vi "Define Columns.vi"() -> (2 "Column Definitions":T1[](array[typedef]) {"MinWidth" min=2 step=1; "AutoSizeMode" items=["None"=1, "ColumnHeader"=2, "AllCellsExceptHeader"=4, "AllCells"=6, "DisplayedCellsExceptHeader"=8, "DisplayedCells"=10, "Fill"=16]; "FillWeight" min=1 max=100})   [LabVIEW 2013, in "Modbus Module editor node.lvclass"]
uses:
  Modbus Module editor node.lvclass
  <vilib>/NI/DCAF Table API/Column/Column Descriptor.ctl
  <vilib>/NI/DCAF Table API/Column/Column Type.ctl
  <vilib>/NI/Tag Bus/tag/Data Type.ctl
  <vilib>/NI/DCAF Table API/Table Manager/Call Back Ref Type Def.ctl
  <vilib>/NI/DCAF/Tag Editor Core/Configuration Editor/Classes/Engine Parent/Engine Parent Editor Node.lvclass
  <vilib>/NI/DCAF/Tag Editor Core/Configuration Editor/Classes/Module editor node/module editor node.lvclass
  <vilib>/NI/DCAF Table API/Column/Column.lvclass
  <vilib>/NI/DCAF Table API/Mapping Column/Mapping Column.lvclass
  <vilib>/NI/DCAF Table API/String Column/String Column.lvclass
  <vilib>/NI/Tag Bus/tag/tag descriptor.lvclass
  <vilib>/NI/DCAF Table API/Table Manager/Table Manager.lvclass
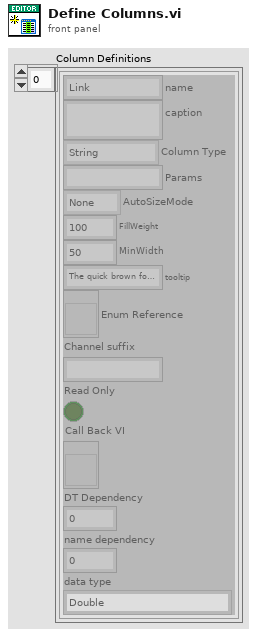
[diagram p1: front panel]
types:
  T1 = typedef "Table Manager.lvlib/Column.lvclass/Column Descriptor.ctl" = cluster{"name":string, "caption":string, "Column Type":T2, "Params":string, "AutoSizeMode":i32, "FillWeight":sgl, "MinWidth":u32, "tooltip":string, "Enum Reference":refnum<vi>, "Channel suffix":string, "Read Only":bool, "Call Back VI":T3, "DT Dependency":i32, "name dependency":i32, "data type":T4}
  T2 = typedef "Table Manager.lvlib/Column.lvclass/Column Type.ctl" = enum16{"String", "Mapping", "Channel Name", "Tag", "Enum", "Data Type", "Numeric"}
  T3 = typedef "Table Manager.lvlib/Table Manager.lvclass/Call Back Ref Type Def.ctl" = refnum<vi>
  T4 = typedef "tag bus.lvlib/tag descriptor.lvclass/Data Type.ctl" = enum16{"Double", "Single", "I64", "I32", "I16", "I8", "U64", "U32", "U16", "U8", "Boolean", "String", "Array of Double", "Array of Single", "Array of I64", "Array of I32", "Array of I16", "Array of I8", "Array of U64", "Array of U32", "Array of U16", "Array of U8", "Array of Boolean", "Array of String"}
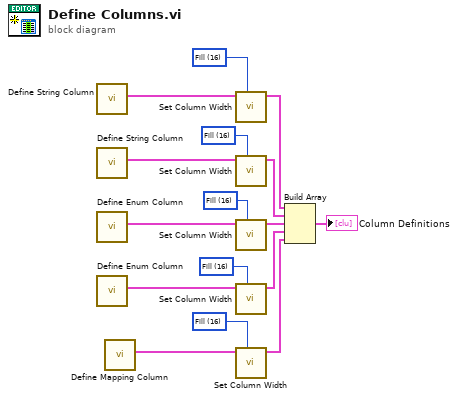
[diagram p0: block diagram]
diagram:
  w1 = 16 items=["None"=1, "ColumnHeader"=2, "AllCellsExceptHeader"=4, "AllCells"=6, "DisplayedCellsExceptHeader"=8, "DisplayedCells"=10, "Fill"=16] ("AutoSizeMode")
  w2 = 16 items=["None"=1, "ColumnHeader"=2, "AllCellsExceptHeader"=4, "AllCells"=6, "DisplayedCellsExceptHeader"=8, "DisplayedCells"=10, "Fill"=16] ("AutoSizeMode")
  w3 = 16 items=["None"=1, "ColumnHeader"=2, "AllCellsExceptHeader"=4, "AllCells"=6, "DisplayedCellsExceptHeader"=8, "DisplayedCells"=10, "Fill"=16] ("AutoSizeMode")
  w4 = 16 items=["None"=1, "ColumnHeader"=2, "AllCellsExceptHeader"=4, "AllCells"=6, "DisplayedCellsExceptHeader"=8, "DisplayedCells"=10, "Fill"=16] ("AutoSizeMode")
  w5 = 16 items=["None"=1, "ColumnHeader"=2, "AllCellsExceptHeader"=4, "AllCells"=6, "DisplayedCellsExceptHeader"=8, "DisplayedCells"=10, "Fill"=16] ("AutoSizeMode")
  n1 = call <vilib>:"Define String Column.vi"() -> ("Table Manager.lvlib:Column.lvclass:Column Descriptor"=w10:T1)  [unwired: 11 in]
  n2 = call <vilib>:"Define String Column.vi"() -> ("Table Manager.lvlib:Column.lvclass:Column Descriptor"=w9:T1)  [unwired: 11 in]
  n3 = call <vilib>:"Define Enum Column.vi"() -> ("Table Manager.lvlib:Column.lvclass:Column Descriptor"=w8:T1)  [unwired: 11 in]
  n4 = call <vilib>:"Define Enum Column.vi"() -> ("Table Manager.lvlib:Column.lvclass:Column Descriptor"=w6:T1)  [unwired: 11 in]
  n5 = call <vilib>:"Define Mapping Column.vi"() -> ("Table Manager.lvlib:Column.lvclass:Column Descriptor"=w7:T1)  [unwired: 11 in]
  n6 = call <vilib>:"Set Column Width.vi"("AutoSizeMode"=w5, "Column Descriptor in"=w10) -> ("Column Descriptor out"=w16:T1)  [unwired: 9 in]
  n7 = call <vilib>:"Set Column Width.vi"("AutoSizeMode"=w4, "Column Descriptor in"=w9) -> ("Column Descriptor out"=w14:T1)  [unwired: 9 in]
  n8 = call <vilib>:"Set Column Width.vi"("AutoSizeMode"=w3, "Column Descriptor in"=w8) -> ("Column Descriptor out"=w13:T1)  [unwired: 9 in]
  n9 = call <vilib>:"Set Column Width.vi"("AutoSizeMode"=w2, "Column Descriptor in"=w6) -> ("Column Descriptor out"=w12:T1)  [unwired: 9 in]
  n10 = call <vilib>:"Set Column Width.vi"("AutoSizeMode"=w1, "Column Descriptor in"=w7) -> ("Column Descriptor out"=w11:T1)  [unwired: 9 in]
  n11 = Build Array(w16, w14, w13, w12, w11) -> (→"Column Definitions":T1[])
